vi "FTW-Messenger-NewObserver.vi"(0 "Messenger":refnum<class "FTW-Messenger.lvclass">, 11 "error in":errorcluster) -> (4 "Messenger out":refnum<class "FTW-Messenger.lvclass">, 6 "Message":refnum<event-registration>, 15 "error out":errorcluster)   [LabVIEW 2013, in "FTW-Messenger.lvclass"]
uses:
  FTW-Messenger.lvclass
  Message/FTW-Message.lvclass
  FTW-Messenger.lvclass/FTW-Messenger.ctl
panel:
  # "Inputs"
  # "Outputs"
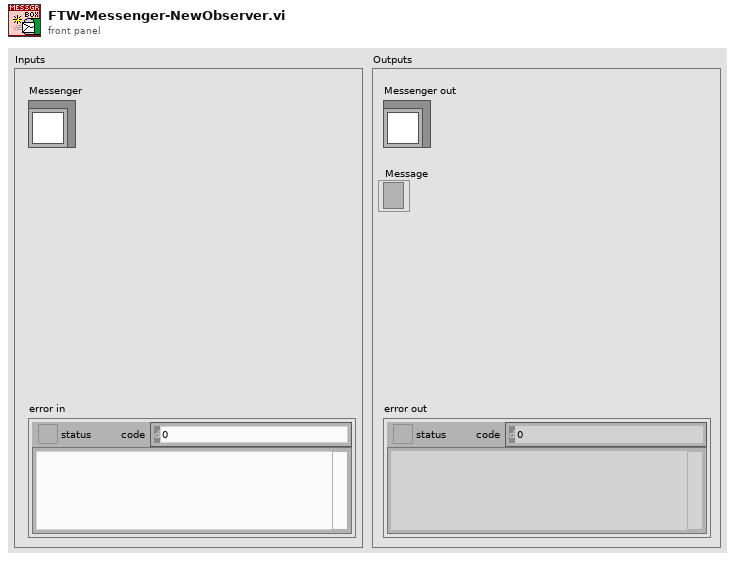
[diagram p1: front panel]
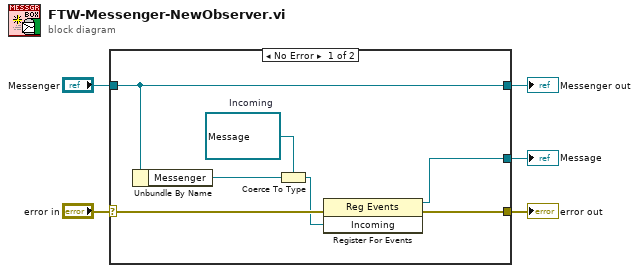
[diagram p0: block diagram]
diagram:
  n1 = case shown="No Error" "error in" {
    selector: "error in" -> [w11 w14]
    tunnel: [w10 w14] -> w3
    tunnel: [w12 w13] -> w4
    tunnel: "Messenger" -> [w12 w13]
    tunnel: [w9 _] -> w1
    frame No Error {
      w6 = refnum<user-event> refnum  # Incoming
      n2 = Unbundle By Name(w12) -> ("Messenger"=w8:refnum<user-event>)
      n3 = Coerce To Type(0:w8, 1:w6) -> (2:w7:refnum<user-event>)
      n4 = register-events(error in=w11, w7) -> (reference out=w9:refnum<event-registration>, error out=w10:errorcluster)  [unwired: 1 in]
    }
    frame Error {
    }
  }
  "Messenger out" <- w4
  "error out" <- w3
  "Message" <- w1
